vi "DefaultFromIni.vi"(8 "error in (no error)":errorcluster, 11 "C37.118 PMU in":refnum<class "C37.118 PMU.lvclass">) -> (0 "error out":errorcluster, 3 "C37.118 PMU out":refnum<class "C37.118 PMU.lvclass">)   [LabVIEW 2018, in "SensorPlugins.lvlib" / "C37.118 PMU.lvclass"]
uses:
  C37.118 PMU.lvclass
  C:/Program Files/National Instruments/LabVIEW 2018/user.lib/NIST/BaseClasses/BasePlugin_class/BasePlugin.lvclass
  Typedef/PMUComms.ctl
  Typedef/eCommsType.ctl
  <userlib>/NIST/BaseClasses/BasePlugin_class/BasePlugin.lvclass/BasePlugin.ctl
  C37.118 PMU.lvclass/C37.118 PMU.ctl
  Accessors/Write PMUComms.vi
  <userlib>/NIST/BaseClasses/BasePlugin_class/Accessors/Read PluginIniFilePath.vi
  Accessors/Read PMUComms.vi
  <vilib>/Utility/error.llb/Error Cluster From Error Code.vi
  PmuBaseClass/PmuBase.lvclass
  <vilib>/ErrorRing/Error Ring.xnode
  <vilib>/Utility/config.llb/NI_LVConfig.lvlib
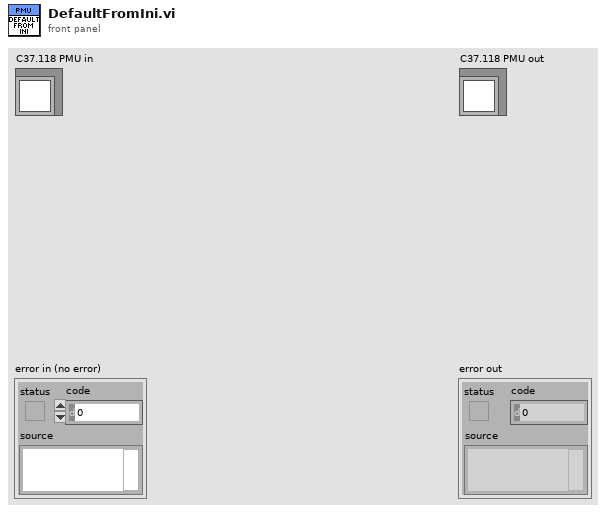
[diagram p1: front panel]
types:
  T1 = typedef "SensorPlugins.lvlib/C37.118 PMU.lvclass/PMUComms.ctl" = cluster{"PMU IP Address":string, "CMD Comms Type":T2, "Data Comms Type":T2, "CMD Port":u16, "Data Port":u16, "PMU ID":u16}
  T2 = typedef "SensorPlugins.lvlib/C37.118 PMU.lvclass/eCommsType.ctl" = enum16{"TCP", "UDP", "USB", "GPIB"}
  T3 = typedef "NI_LVConfig.lvlib/Config Data RefNum.ctl" = refnum<k1>
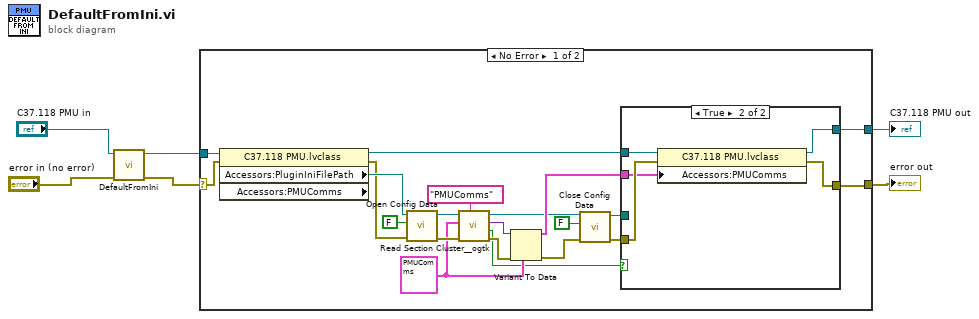
[diagram p0: block diagram]
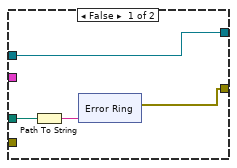
[diagram p2: hidden frame]
diagram:
  n1 = call-parent "DefaultFromIni.vi"("error in (no error)"="error in (no error)", "PmuBase in"="C37.118 PMU in") -> ("error out"=w4:errorcluster, "PmuBase out"=w2:refnum<class "C37.118 PMU.lvclass">)  [unwired: 8 in]
  n2 = case shown="No Error" w4 {
    selector: w4 -> [w26 w45]
    tunnel: [w11 w45] -> w3
    tunnel: w2 -> [w27 w44]
    tunnel: [w12 w44] -> w1
    frame No Error {
      w18 = T1 {"PMU IP Address"="192.92.92.92", "CMD Comms Type"=enum."TCP", "Data Comms Type"=enum."TCP", "CMD Port"=4712, "Data Port"=4712, "PMU ID"=1} ("PMU Comms")
      n3 = property class="C37.118 PMU.lvclass" props=["Accessors:PluginIniFilePath", "Accessors:PMUComms"](reference=w27, error in=w26) -> (reference out=w16:refnum<class "C37.118 PMU.lvclass">, error out=w23:errorcluster, "Accessors:PluginIniFilePath"=w25:path)  [unwired: 1 out]
      n4 = call <vilib>:"Open Config Data.vi"("error in (no error)"=w23, "create file if necessary (T)"=FALSE, "configuration file path"=w25) -> ("error out"=w22:errorcluster, "refnum"=w21:T3)  [unwired: 6 in, 1 out]
      n5 = call <userlib>:"Read Section Cluster__ogtk.vi"("section (optional)"="PMUComms", "error in (no error)"=w22, "Section Formatted Cluster Type"=w18, "refnum"=w21) -> ("error out"=w17:errorcluster, "all found?"=w15:bool, "Section Formatted Cluster"=w19:variant, "dup refnum"=w9:T3)  [unwired: 3 in, 1 out]
      n6 = Variant To Data(error in=w17, type=w18, Variant=w19) -> (data=w13:T1, error out=w7:errorcluster)
      n7 = call <vilib>:"Close Config Data.vi"("error in (no error)"=w7, "write file if changed (T)"=FALSE, "refnum"=w9) -> ("error out"=w14:errorcluster, "file path"=w10:path)  [unwired: 7 in]
      n8 = case shown="True" w15 {
        tunnel: w16 -> [w28 w43]
        tunnel: w14 -> [_ w42]
        tunnel: w13 -> [_ w41]
        tunnel: [w28 w40] -> w12
        tunnel: [w29 w39] -> w11
        tunnel: w10 -> [w31 _]
        frame False {
          n9 = Path To String(path=w31) -> (string=w30:string)
          n10 = xnode "Error Ring"("parameter 0"=w30) -> ("error out"=w29:errorcluster)
        }
        frame True {
          n11 = property class="C37.118 PMU.lvclass"(reference=w43, error in=w42, "Accessors:PMUComms"=w41) -> (reference out=w40:refnum<class "C37.118 PMU.lvclass">, error out=w39:errorcluster)
        }
      }
    }
    frame Error {
    }
  }
  "error out" <- w3
  "C37.118 PMU out" <- w1
